vi "WPI_CounterReset.vi"(8 "error in (no error)":errorcluster, 11 "CounterDevRef in":T1) -> (0 "error out":errorcluster, 3 "CounterDevRef out":T1)   [LabVIEW 2017]
doc: "Resets the counter you specify to 0.\n\nThis software is licensed. Open the labview\\readme\\WPI Robotics Library Open Source License.txt file for more information."
uses:
  <vilib>/Rock Robotics/WPI/Counter/WPI_CounterDevRef.ctl
  <vilib>/Rock Robotics/SystemInterfaces/Counter/FPGA_CounterCtrSystemIndex.ctl
  <vilib>/Rock Robotics/SystemInterfaces/Counter/FPGA_CounterERRInvalidResource.vi
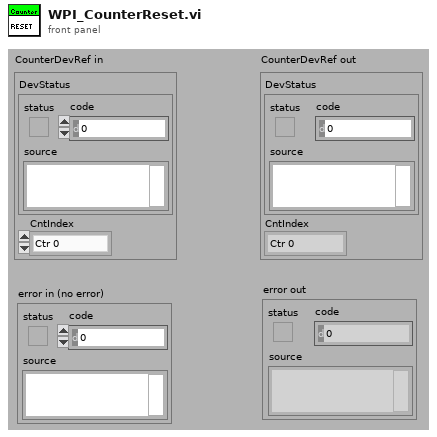
[diagram p1: front panel]
types:
  T1 = typedef "WPI_CounterDevRef.ctl" = cluster{"DevStatus":errorcluster, "CntIndex":T2}
  T2 = typedef "FPGA_CounterCtrSystemIndex.ctl" = enum8{"Ctr 0", "Ctr 1", "Ctr 2", "Ctr 3", "Ctr 4", "Ctr 5", "Ctr 6", "Ctr 7", "Invalid"}
  T3 = typedef "FPGA_CounterCtrDevRef.ctl" = cluster{"DevStatus":errorcluster, "CntIndex":T2}
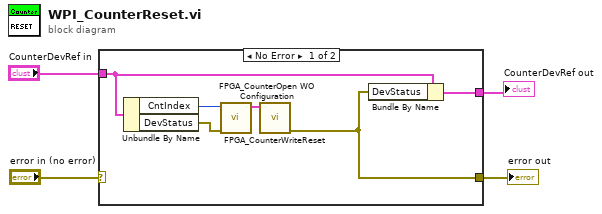
[diagram p0: block diagram]
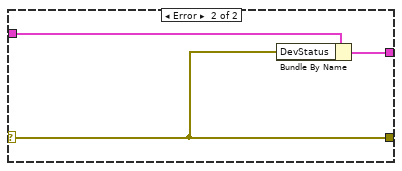
[diagram p2: hidden frame]
diagram:
  n1 = case shown="No Error" "error in (no error)" {
    selector: "error in (no error)" -> [_ w11]
    tunnel: "CounterDevRef in" -> [w9 w13]
    tunnel: [w8 w12] -> w3
    tunnel: [w5 w11] -> w1
    frame No Error {
      n2 = Unbundle By Name(w9) -> ("CntIndex"=w6:T2, "DevStatus"=w7:errorcluster)
      n3 = call <vilib>:"FPGA_CounterOpen WO Configuration.vi"("error in"=w7, "CntIndex"=w6) -> ("Ctr Ref"=w10:T3)  [unwired: 1 in, 8 out]
      n4 = call <vilib>:"FPGA_CounterWriteReset.vi"("Ctr Ref in"=w10) -> ("error out"=w5:errorcluster)  [unwired: 2 in, 8 out]
      n5 = Bundle By Name(cluster=w9, "DevStatus"=w5) -> (w8:T1)
    }
    frame Error {
      n6 = Bundle By Name(cluster=w13, "DevStatus"=w11) -> (w12:T1)
    }
  }
  "CounterDevRef out" <- w3
  "error out" <- w1
